vi "LabVIEWTempLogger_USB-TC.vi"() -> ()   [LabVIEW 2010]
uses:
  Instance           1 25Saved   LabVIEWTempLogger .vi
  Instance           3 25Saved   LabVIEWTempLogger .vi
  Instance           2 25Saved   LabVIEWTempLogger .vi
panel:
  in  "Log Data?":bool=TRUE
  in  "File Path":path=path "C:/Users/Public/Documents/log.lvm" caption="Filename"
  out "Current Reading":dbl format="%#.1g"
  in  "Description":string="Enter a description"
  in  "Stop":bool
  out "Waveform Chart":dynamicdata(graph)=[{"t0"=timestamp(3340208761.0542846 s since 1904-01-01), "dt"=1.0, "Y"=[-166.57635028815426], "attributes"=variant("NI_ChannelName"=variant(string "Temperature"), "NI_UnitDescription"=variant(string "Deg C"))}]
  # "NI USB-TC01 LabVIEW Temperature Logger"
  # "Switch to the block diagram (Window » Show Block Diagram) to configure the device, thermocouple type, and temperature unit."
  # "© 2010 National Instruments. All rights reserved."
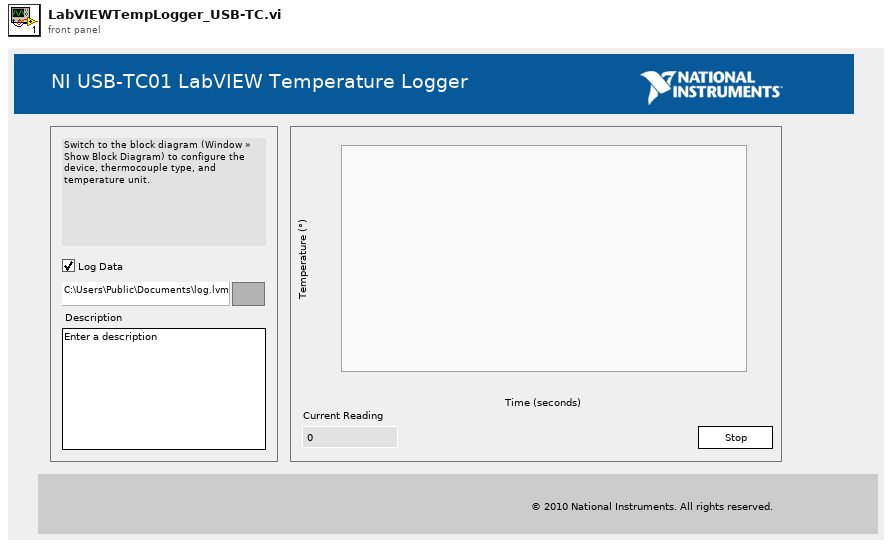
[diagram p1: front panel]
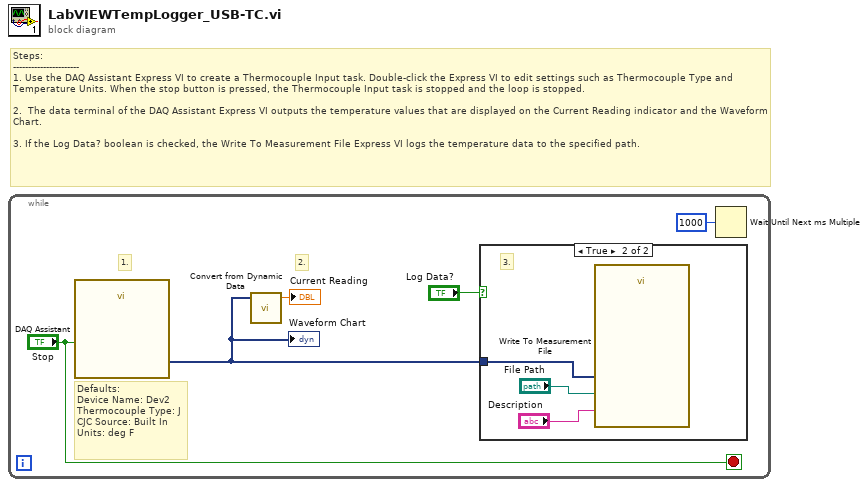
[diagram p0: block diagram]
diagram:
  # "Steps:\n----------------------\n1. Use the DAQ Assistant Express VI to create a Thermocouple Input task. Double-click the Express VI to edit settings such as Thermocouple Type and Temperature Units. When the stop button is pressed, the Thermocouple Input task is stopped and the loop is stopped.\n\n2.  The data terminal of the DAQ Assistant Express VI outputs the temperature values that are displayed on the Current Reading indicator and the Waveform Chart.\n\n3. If the Log Data? boolean is checked, the Write To Measurement File Express VI logs the temperature data to the specified path."
  n1 = while {
    stop <- "Stop" stop-if-true
    # "Defaults:\nDevice Name: Dev2\nThermocouple Type: J\nCJC Source: Built In\nUnits: deg F"
    # "2."
    # "1."
    n2 = call "DAQ Assistant"("stop (T)"="Stop") -> ("data"=w4:dynamicdata)  [unwired: 16 in, 2 out]
    "Waveform Chart" <- w4
    n3 = call "Convert from Dynamic Data"("Dynamic Data Type"=w4) -> ("Scalar"=→"Current Reading":dbl)  [unwired: 3 in]
    n4 = case shown="True" "Log Data?" {
      tunnel: w4 -> [_ w7]
      frame False {
      }
      frame True {
        # "3."
        n5 = call "Write To Measurement File"("Signals"=w7, "Filename"="File Path", "Comment"="Description") -> ()  [unwired: 14 in, 3 out]
      }
    }
    n6 = Wait Until Next ms Multiple(millisecond multiple=u32 1000) -> ()  [unwired: 1 out]
  }
